vi "PXI-AI Data Bank.vi"(7 "Action":T1, 8 "error in (no error)":errorcluster, 11 "Data In":dbl[][](array[numeric])) -> (0 "error out":errorcluster, 3 "Data Out":dbl[][](array[numeric]))   [LabVIEW 2020]
uses:
  Type Defs/PXI-DO Signal Bank Action.ctl
  PXI Globals.vi
panel:
  out "Waveform Graph":dbl[][](graph)
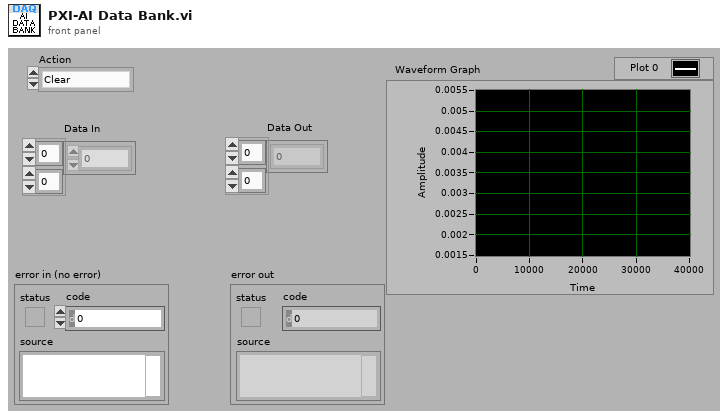
[diagram p1: front panel]
types:
  T1 = typedef "PXI-DO Signal Bank Action.ctl" = enum16{"Clear", "Write", "Read"}
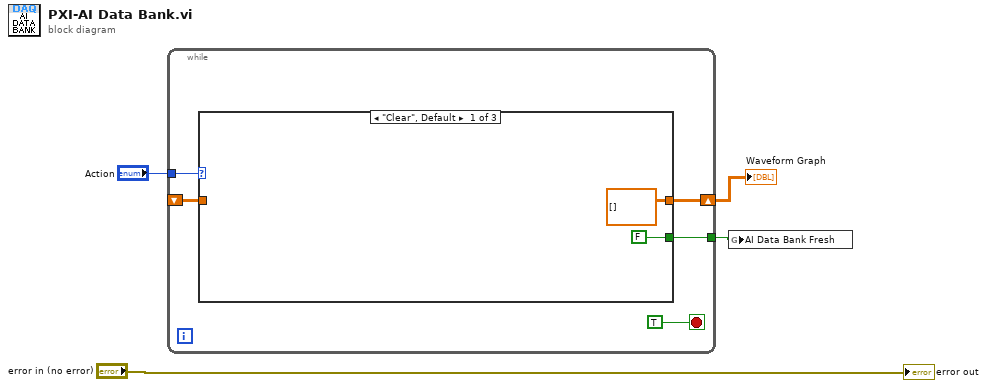
[diagram p0: block diagram]
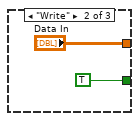
[diagram p2: hidden frame]
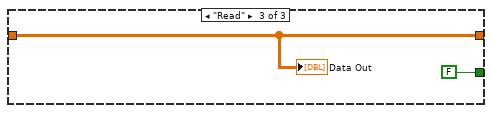
[diagram p3: hidden frame]
diagram:
  n1 = while {
    tunnel: "Action" -> [w8]
    shift-right: [w6] -> w2
    shift-left: _ -> [w7]
    tunnel: [w5] -> w3
    stop <- TRUE stop-if-true
    n2 = case shown="\"Clear\", Default" w8 {
      tunnel: [dbl[][] [] ("Data In") "Data In" w14] -> w6
      tunnel: w7 -> [_ _ w14]
      tunnel: [FALSE TRUE FALSE] -> w5
      frame "Clear", Default {
      }
      frame "Write" {
      }
      frame "Read" {
        "Data Out" <- w14
      }
    }
  }
  "Waveform Graph" <- w2
  n3 = global write "PXI Globals.vi" "AI Data Bank Fresh"(w3) -> ()
  "error out" <- "error in (no error)"
